vi "Configure First and Last Packet Data Type Select.vi"(0 "fpga interface in":refnum<k20>, 5 "first packet data type select":T1, 7 "last packet data type select":T1, 9 "first and last packet virtual channel must match (T)":bool=TRUE, 11 "error in (no error)":errorcluster, 12 "enable first and last packet select":bool, 13 "stop timeout (s)":dbl=1.0) -> (4 "fpga interface out":refnum<k20>, 15 "error out":errorcluster)   [LabVIEW 2023, in "GettingStarted_Acq_148X_Host.lvlib"]
uses:
  GettingStarted_Acq_148X_Host.lvlib
  <instrlib>/FlexRIO/CSI-2/v2/Common/Types/LLP Data Type.ctl
  Types/148x_Acq_FPGA_Reference.ctl
  0828d4c4-e074-4f11-89cd-788a20bfe090.vi
  72a8fd79-fec7-4a4d-8516-91c839b9c0be.vi
  <vilib>/Utility/error.llb/Error Cluster From Error Code.vi
  <vilib>/rvi/errors/niLvFpgaAdjustHostInterfaceError.vi
  <vilib>/rvi/interface/nirviReadWriteControl/nirviReadWriteControl.xnode
  <instrlib>/FlexRIO/CSI-2/v2/Host/NI CSI-2 API Host v2.lvlib
  <vilib>/rvi/interface/Simulation/niFpgaSimulationCallBeginRW.vi
  NiFpgaLv.dll
  <instrlib>/FlexRIO/CSI-2/v2/Common/NI CSI-2 API Common v2.lvlib
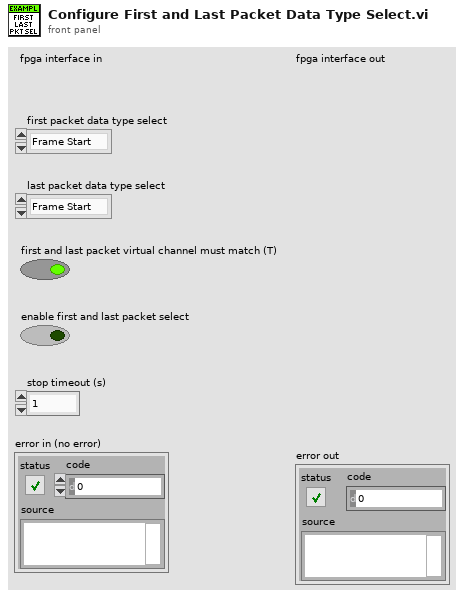
[diagram p1: front panel]
types:
  T1 = typedef "NI CSI-2 API Common v2.lvlib/LLP Data Type.ctl" = enum8{"Frame Start", "Frame End", "Line Start", "Line End", "End of Transmission", "Reserved 0", "Reserved 1", "Reserved 2", "Generic Short Packet 1", "Generic Short Packet 2", "Generic Short Packet 3", "Generic Short Packet 4", "Generic Short Packet 5", "Generic Short Packet 6", "Generic Short Packet 7", "Generic Short Packet 8", "Null", "Blanking Data", "Embedded 8-bit non Image Data", "Generic Long Packet 1", "Generic Long Packet 2", "Generic Long Packet 3", "Generic Long Packet 4", "Reserved 3", "YUV420 8-bit", "YUV420 10-bit", "Legacy YUV420 8-bit", "Reserved 4", "YUV420 8-bit Chroma Shifted", "YUV420 10-bit Chroma Shifted", "YUV422 8-bit", "YUV422 10-bit", "RGB444", "RGB555", "RGB565", "RGB666", "RGB888", "Reserved 5", "Reserved 6", "RAW 24", "RAW 6", "RAW 7", "RAW 8", "RAW 10", "RAW 12", "RAW 14", "RAW 16", "RAW 20", "User Defined 8-bit Data 1", "User Defined 8-bit Data 2", "User Defined 8-bit Data 3", "User Defined 8-bit Data 4", "User Defined 8-bit Data 5", "User Defined 8-bit Data 6", "User Defined 8-bit Data 7", "User Defined 8-bit Data 8", "USL Command", "Reserved 7", "Reserved 8", "Reserved 9", "Reserved 10", "Reserved 11", "Reserved 12", "LRTE EPD Spacer"}
  T2 = typedef "GettingStarted_Acq_148X_Host.lvlib/148x_Acq_FPGA_Reference.ctl" = refnum<k20>
  T3 = cluster{"channel acq config":cluster{"stop timeout (cycles)":u32, "first packet data type select mask":u64, "last packet data type select mask":u64, "first and last packet virtual channel must match":bool}, "virtual channel packet filter mask":u16, "data type packet filter mask":u64, "select corrected csi-2 data":bool, "enable channel":bool}[]
  T4 = cluster{"channel acq config":cluster{"stop timeout (cycles)":u32, "first packet data type select mask":u64, "last packet data type select mask":u64, "first and last packet virtual channel must match":bool}, "virtual channel packet filter mask":u16, "data type packet filter mask":u64, "select corrected csi-2 data":bool, "enable channel":bool}
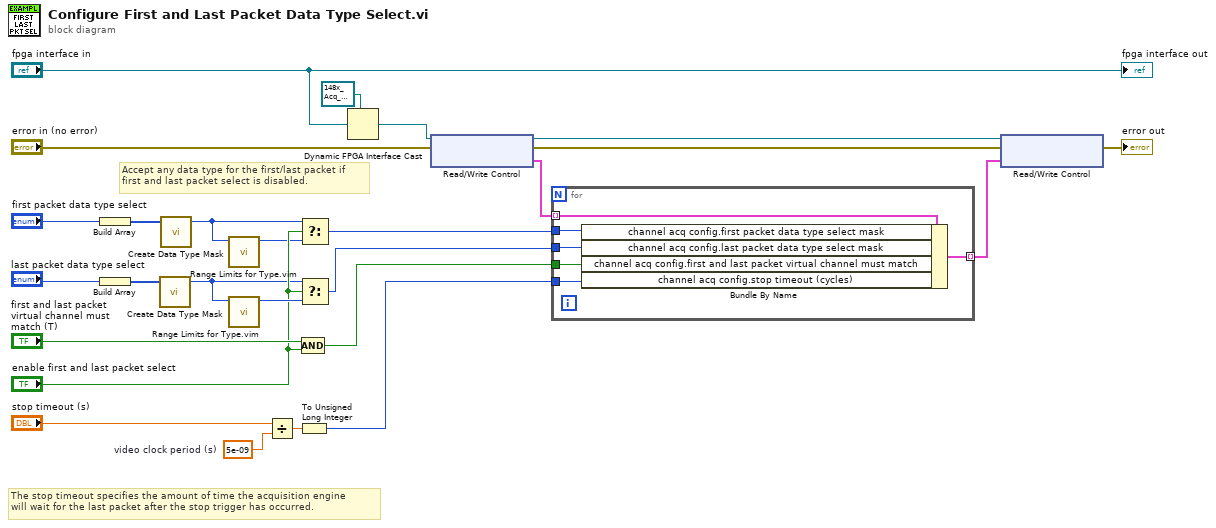
[diagram p0: block diagram]
diagram:
  w22 = 5e-09  # video clock period (s)
  # "The stop timeout specifies the amount of time the acquisition engine \nwill wait for the last packet after the stop trigger has occurred."
  # "Accept any data type for the first/last packet if \nfirst and last packet select is disabled."
  n1 = Build Array("first packet data type select") -> (w20:T1[])
  n2 = Build Array("last packet data type select") -> (w18:T1[])
  n3 = call <instrlib>:"Create Data Type Mask.vi"("data types"=w18) -> ("data type mask"=w14:u64)  [unwired: 4 in]
  n4 = call <instrlib>:"Create Data Type Mask.vi"("data types"=w20) -> ("data type mask"=w12:u64)  [unwired: 4 in]
  n5 = call "Range Limits for Type.vim"("type"=w12) -> ("maximum value for type"=w13:u64)  [unwired: 9 in, 1 out]
  n6 = call "Range Limits for Type.vim"("type"=w14) -> ("maximum value for type"=w16:u64)  [unwired: 9 in, 1 out]
  n7 = Divide(x="stop timeout (s)", y=w22) -> (x/y=w23:dbl)
  n8 = To Unsigned Long Integer(number=w23) -> (unsigned 32bit integer=w7:u32)
  n9 = Select(t=w12, s="enable first and last packet select", f=w13) -> (s? t:f=w4:u64)
  n10 = Select(t=w14, s="enable first and last packet select", f=w16) -> (s? t:f=w5:u64)
  n11 = Compound Arithmetic op=AND("first and last packet virtual channel must match (T)", "enable first and last packet select") -> (w6:bool)
  n12 = Dynamic FPGA Interface Cast(Session In=T2 refnum ("FPGA VI Reference Out"), Type="fpga interface in") -> (Session Out=w1:T2)
  n13 = xnode "Read/Write Control"("FPGA VI Reference In"=w1, "error in"="error in (no error)") -> ("FPGA VI Reference Out"=w9:T2, "error out"=w10:errorcluster, "channel configs"=w11:T3)
  n14 = for {
    tunnel: w11 -> [w32] mode=indexing
    tunnel: [w31] -> w8 mode=indexing
    tunnel: w7 -> [w30]
    tunnel: w6 -> [w29]
    tunnel: w5 -> [w28]
    tunnel: w4 -> [w27]
    n15 = Bundle By Name(cluster=w32, "channel acq config.first packet data type select mask"=w27, "channel acq config.last packet data type select mask"=w28, "channel acq config.first and last packet virtual channel must match"=w29, "channel acq config.stop timeout (cycles)"=w30) -> (w31:T4)
  }
  n16 = xnode "Read/Write Control"("FPGA VI Reference In"=w9, "error in"=w10, "channel configs"=w8) -> ("error out"=→"error out":errorcluster)  [unwired: 1 out]
  "fpga interface out" <- "fpga interface in"
